vi "INSERT many rows Template code.vi"   [LabVIEW 2011, in "SQLite.lvlib"]
doc: "Code template for inserting many rows in a Table."
uses:
  SQLite.lvlib
  SQL Statement.lvclass
  SQL Connection/Connection.lvclass
  Transaction Helpers/Transaction.lvlib
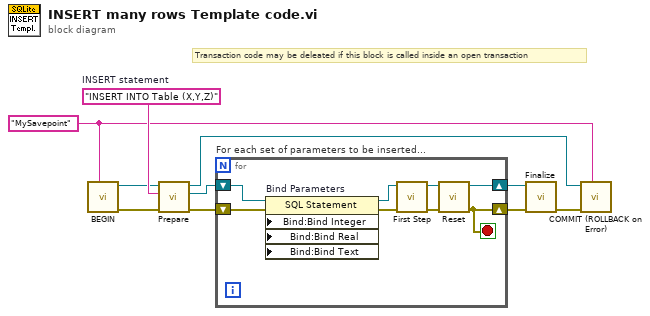
[diagram p0: block diagram]
diagram:
  w3 = "MySavepoint" ("Savepoint name")
  w8 = "INSERT INTO Table (X,Y,Z)"  # INSERT statement
  # "Transaction code may be deleated if this block is called inside an open transaction"
  n1 = call "BEGIN.vi"("Savepoint name"=w3) -> ("error out"=w4:errorcluster, "Connection out"=w5:refnum<class "Connection.lvclass">)  [unwired: 9 in]
  n2 = call "Prepare.vi"("error in (no error)"=w4, "SQL"=w8, "SQLite Connection in"=w5) -> ("error out"=w9:errorcluster, "SQL Statement out"=w10:refnum<class "SQL Statement.lvclass">, "SQLite Connection out"=w2:refnum<class "Connection.lvclass">)  [unwired: 4 in, 2 out]
  n3 = for "For each set of parameters to be inserted..." {
    shift-right: [w12] -> w7
    shift-left: w10 -> [w18]
    shift-right: [w11] -> w6
    shift-left: w9 -> [w15]
    stop <- w11 stop-if-true
    n4 = property on="Bind Parameters" class="SQL Statement" props=["Bind:Bind Integer", "Bind:Bind Real", "Bind:Bind Text"](reference=w18, error in=w15) -> (reference out=w17:refnum<class "SQL Statement.lvclass">, error out=w16:errorcluster)  [unwired: 3 in]
    n5 = call "First Step.vi"("error in (no error)"=w16, "SQL Statement in"=w17) -> ("error out"=w14:errorcluster, "SQL Statement out"=w13:refnum<class "SQL Statement.lvclass">)  [unwired: 7 in, 1 out]
    n6 = call "Reset.vi"("error in (no error)"=w14, "SQL Statement in"=w13) -> ("error out"=w11:errorcluster, "SQL Statement out"=w12:refnum<class "SQL Statement.lvclass">)  [unwired: 8 in]
  }
  n7 = call "Finalize.vi"("error in (no error)"=w6, "SQL Statement in"=w7) -> ("error out"=w1:errorcluster)  [unwired: 9 in]
  n8 = call "COMMIT (ROLLBACK on Error).vi"("Savepoint name"=w3, "error in (no error)"=w1, "Connection in"=w2) -> ()  [unwired: 7 in, 2 out]
